vi "Periodic Tasks.vi"(8 "error in":errorcluster) -> ()   [LabVIEW 2013]
doc: "This VI runs in parallel to other tasks. It can contain as many user-defined periodic loops as you need. These can carry out PID or other sorts of timed response."
uses:
  <vilib>/Rock Robotics/SystemInterfaces/Utilities/FPGA_UtilitiesLED Source.ctl
  <vilib>/Rock Robotics/SystemInterfaces/Utilities/FPGA_UtilitiesLED State.ctl
  <vilib>/Rock Robotics/WPI/DriverStation/DriverStationLCD/WPI_DriverStationLCDLCDLine.ctl
  Robot Global Data.vi
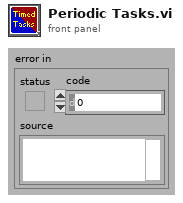
[diagram p1: front panel]
types:
  T1 = typedef "WPI_AnalogChannelDevRef.ctl" = cluster{"DevStatus":errorcluster, "Analog Module":T2, "Analog Channel":T3}
  T2 = typedef "FPGA_TypedefAnalogModule.ctl" = enum16{"Analog Module 1", "Analog Module 2"}
  T3 = typedef "FPGA_AIChannel.ctl" = enum8{"AI 1", "AI 2", "AI 3", "AI 4", "AI 5", "AI 6", "AI 7", "AI 8", "Invalid"}
  T4 = typedef "WPI_DigitalInputDevRef.ctl" = cluster{"DevStatus":errorcluster, "DIO Channel":T5, "Digital Module":T6}
  T5 = typedef "FPGA_DIOChannel.ctl" = enum8{"DIO 1", "DIO 2", "DIO 3", "DIO 4", "DIO 5", "DIO 6", "DIO 7", "DIO 8", "DIO 9", "DIO 10", "DIO 11", "DIO 12", "DIO 13", "DIO 14", "Invalid"}
  T6 = typedef "FPGA_TypedefDigitalModule.ctl" = enum16{"Digital Module 1", "Digital Module 2"}
  T7 = typedef "WPI_EncoderDevRef.ctl" = cluster{"DevStatus":errorcluster, "EncoderIndex":T8, "CounterIndex":T9, "DistancePerCount":dbl, "Decoding Type":T10}
  T8 = typedef "FPGA_EncoderIdx.ctl" = enum8{"Enc 0", "Enc 1", "Enc 2", "Enc 3", "Invalid"}
  T9 = typedef "FPGA_CounterCtrSystemIndex.ctl" = enum8{"Ctr 0", "Ctr 1", "Ctr 2", "Ctr 3", "Ctr 4", "Ctr 5", "Ctr 6", "Ctr 7", "Invalid"}
  T10 = typedef "WPI_EncoderType.ctl" = enum16{"1x", "2x", "4x"}
  T11 = cluster{"Winch Desired Location":dbl, "Winch Desired Location 2":dbl, "Winch Desired Location 3":dbl}
  T12 = typedef "FPGA_UtilitiesLED State.ctl" = enum16{"Off", "On", "Toggle"}
  T13 = typedef "FPGA_UtilitiesLED Source.ctl" = enum16{"User LED", "FPGA LED"}
  T14 = typedef "WPI_DriverStationLCDLCDLine.ctl" = enum16{"Main - Line 1", "User - Line 2", "User - Line 3", "User - Line 4", "User - Line 5", "User - Line 6"}
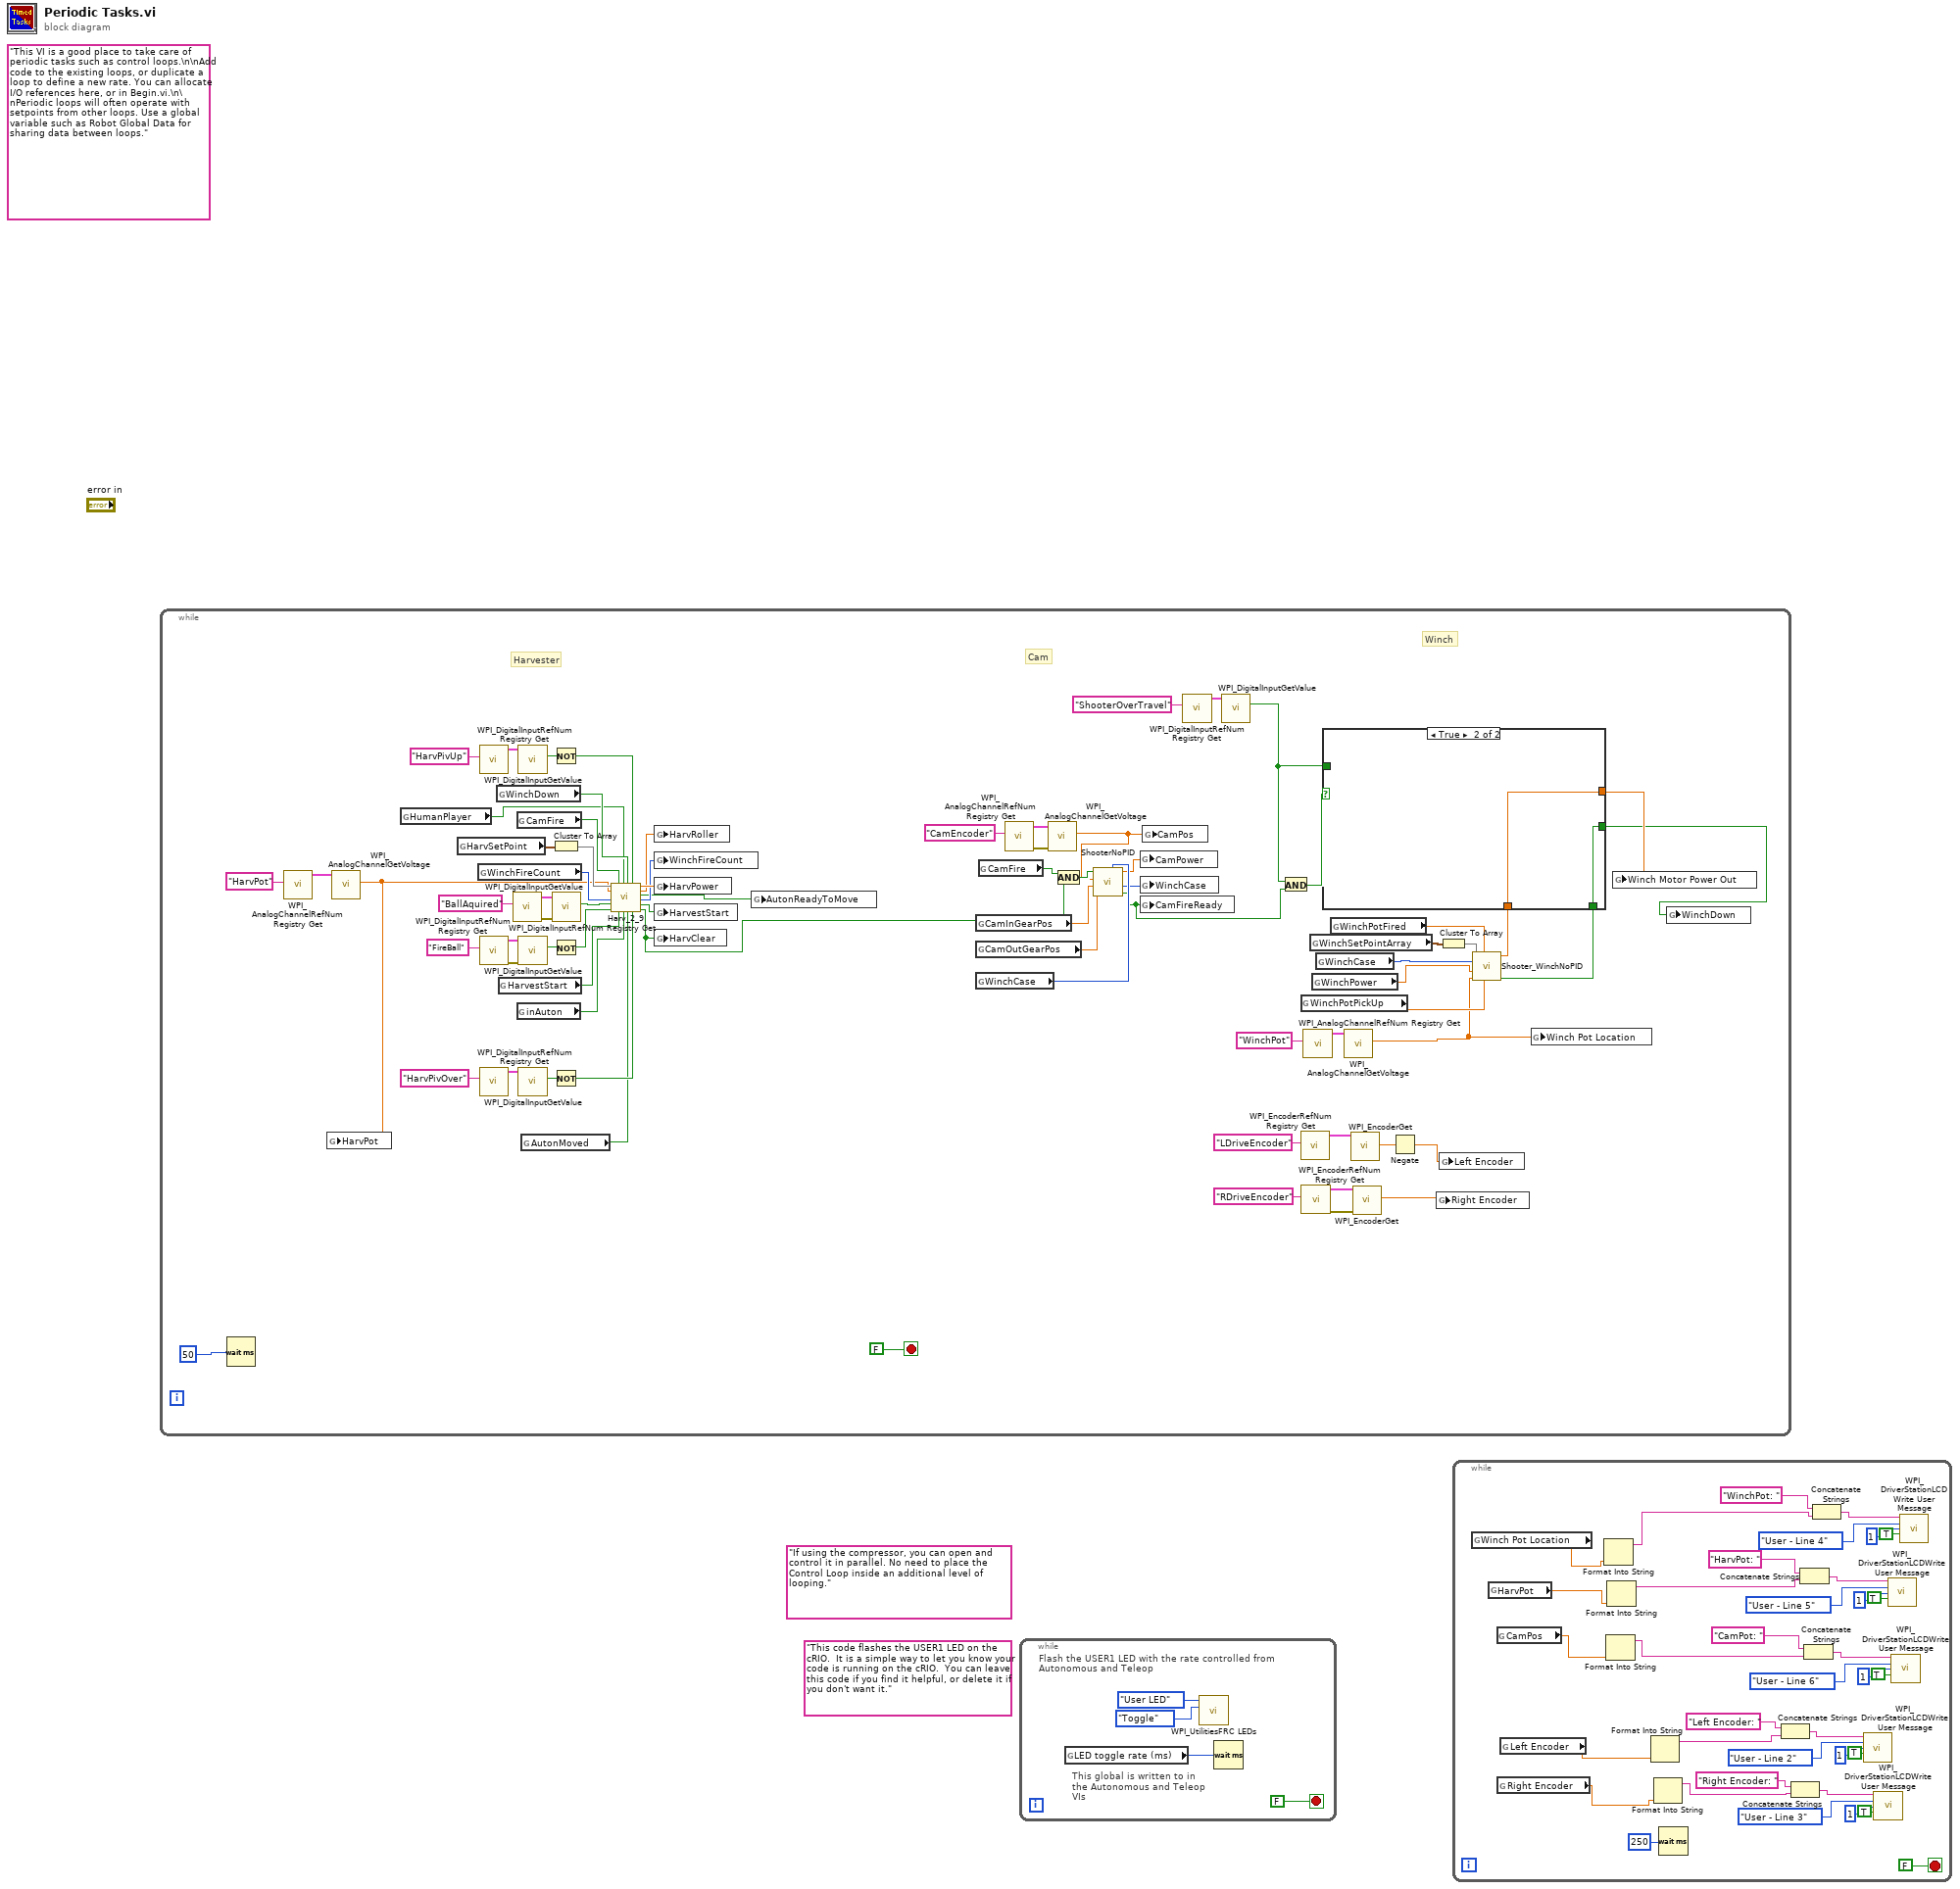
[diagram p0: block diagram]
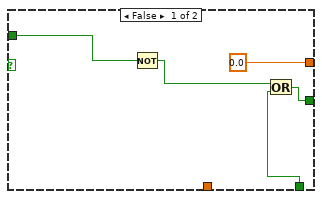
[diagram p2: hidden frame]
diagram:
  (unwired) "If using the compressor, you can open and control it in parallel. No need to place the Control Loop inside an additional level of looping."
  (unwired) "This code flashes the USER1 LED on the cRIO.  It is a simple way to let you know your code is running on the cRIO.  You can leave this code if you find it helpful, or delete it if you don't want it."
  (unwired) "This VI is a good place to take care of periodic tasks such as control loops.\n\nAdd code to the existing loops, or duplicate a loop to define a new rate. You can allocate I/O references here, or in Begin.vi.\n\nPeriodic loops will often operate with setpoints from other loops. Use a global variable such as Robot Global Data for sharing data between loops."
  n1 = while {
    stop <- FALSE stop-if-true
    # "Winch"
    # "Cam"
    # "Harvester"
    n2 = Wait (ms)(milliseconds to wait=u32 50) -> ()  [unwired: 1 out]
    n3 = call <vilib>:"WPI_AnalogChannelRefNum Registry Get.vi"("refnum name"="HarvPot") -> ("AIDeviceRef"=w73:T1)  [unwired: 9 in, 1 out]
    n4 = call <vilib>:"WPI_AnalogChannelGetVoltage.vi"("AIDeviceRef"=w73) -> ("Voltage"=w12:dbl)  [unwired: 8 in, 2 out]
    n5 = global write "Robot Global Data.vi" "HarvPot"(w12) -> ()
    n6 = global read "Robot Global Data.vi" "HumanPlayer"() -> (w3:bool)
    n7 = global read "Robot Global Data.vi" "HarvSetPoint"() -> (w40:cluster{"Out":dbl, "In":dbl, "Clear":dbl})
    n8 = global read "Robot Global Data.vi" "WinchFireCount"() -> (w15:i32)
    n9 = call <vilib>:"WPI_DigitalInputRefNum Registry Get.vi"("refnum name"="HarvPivUp") -> ("DigitalInputDevRef"=w57:T4)  [unwired: 9 in, 1 out]
    n10 = call <vilib>:"WPI_DigitalInputRefNum Registry Get.vi"("refnum name"="FireBall") -> ("error out"=w46:errorcluster, "DigitalInputDevRef"=w47:T4)  [unwired: 9 in]
    n11 = call <vilib>:"WPI_DigitalInputRefNum Registry Get.vi"("refnum name"="HarvPivOver") -> ("DigitalInputDevRef"=w65:T4)  [unwired: 9 in, 1 out]
    n12 = global read "Robot Global Data.vi" "WinchDown"() -> (w33:bool)
    n13 = global read "Robot Global Data.vi" "HarvestStart"() -> (w44:bool)
    n14 = call <vilib>:"WPI_DigitalInputRefNum Registry Get.vi"("refnum name"="BallAquired") -> ("error out"=w53:errorcluster, "DigitalInputDevRef"=w52:T4)  [unwired: 9 in]
    n15 = global read "Robot Global Data.vi" "CamFire"() -> (w45:bool)
    n16 = global read "Robot Global Data.vi" "inAuton"() -> (w17:bool)
    n17 = call <vilib>:"WPI_DigitalInputGetValue.vi"("DigitalInputDevRef"=w57) -> ("Value"=w36:bool)  [unwired: 8 in, 2 out]
    n18 = call <vilib>:"WPI_DigitalInputGetValue.vi"("error in (no error)"=w46, "DigitalInputDevRef"=w47) -> ("Value"=w43:bool)  [unwired: 7 in, 2 out]
    n19 = call <vilib>:"WPI_DigitalInputGetValue.vi"("DigitalInputDevRef"=w65) -> ("Value"=w38:bool)  [unwired: 8 in, 2 out]
    n20 = global read "Robot Global Data.vi" "AutonMoved"() -> (w2:bool)
    n21 = Not(x=w36) -> (.not. x?=w35:bool)
    n22 = Cluster To Array(cluster=w40) -> (array=w39:dbl[])
    n23 = call <vilib>:"WPI_DigitalInputGetValue.vi"("error in (no error)"=w53, "DigitalInputDevRef"=w52) -> ("Value"=w42:bool)  [unwired: 7 in, 2 out]
    n24 = Not(x=w43) -> (.not. x?=w41:bool)
    n25 = Not(x=w38) -> (.not. x?=w37:bool)
    n26 = call "Harv_2_9.vi"("HarvSetpoints"=w39, "HarvPot"=w12, "Count"=w15, "BallAcquired"=w42, "FireBallSen"=w41, "Fire"=w45, "Harvest"=w44, "HPButton"=w3, "inAuton?"=w17, "WinchDown"=w33, "AutonMoved"=w2, "HarvPivUP"=w35, "HarvPivPickupLim"=w37) -> ("HarvPower"=w50:dbl, "HarvRoller"=w49:dbl, "AutonReadyToMove"=w1:bool, "CountOut"=w14:i32, "HarvStart"=w34:bool, "HarvCleared"=w7:bool)  [unwired: 1 in]
    n27 = global write "Robot Global Data.vi" "HarvRoller"(w49) -> ()
    n28 = global write "Robot Global Data.vi" "WinchFireCount"(w14) -> ()
    n29 = global write "Robot Global Data.vi" "HarvPower"(w50) -> ()
    n30 = global write "Robot Global Data.vi" "HarvestStart"(w34) -> ()
    n31 = global write "Robot Global Data.vi" "HarvClear"(w7) -> ()
    n32 = global write "Robot Global Data.vi" "AutonReadyToMove"(w1) -> ()
    n33 = global read "Robot Global Data.vi" "CamInGearPos"() -> (w22:dbl)
    n34 = global read "Robot Global Data.vi" "CamOutGearPos"() -> (w21:dbl)
    n35 = global read "Robot Global Data.vi" "WinchCase"() -> (w23:i32)
    n36 = global read "Robot Global Data.vi" "CamFire"() -> (w59:bool)
    n37 = call <vilib>:"WPI_AnalogChannelRefNum Registry Get.vi"("refnum name"="CamEncoder") -> ("error out"=w61:errorcluster, "AIDeviceRef"=w60:T1)  [unwired: 9 in]
    n38 = call <vilib>:"WPI_AnalogChannelGetVoltage.vi"("error in (no error)"=w61, "AIDeviceRef"=w60) -> ("Voltage"=w11:dbl)  [unwired: 7 in, 2 out]
    n39 = And(x=w59, y=w7) -> (x .and. y?=w24:bool)
    n40 = call "ShooterNoPID.vi"("WinchCaseIn"=w23, "InGearPosLow"=w21, "InGearPosHigh"=w22, "Pot"=w11, "Fire"=w24) -> ("There?"=w18:bool, "WinchCase"=w19:i32, "Power"=w20:dbl)  [unwired: 4 in]
    n41 = global write "Robot Global Data.vi" "CamPower"(w20) -> ()
    n42 = global write "Robot Global Data.vi" "WinchCase"(w19) -> ()
    n43 = global write "Robot Global Data.vi" "CamFireReady"(w18) -> ()
    n44 = global write "Robot Global Data.vi" "CamPos"(w11) -> ()
    n45 = call <vilib>:"WPI_DigitalInputRefNum Registry Get.vi"("refnum name"="ShooterOverTravel") -> ("DigitalInputDevRef"=w56:T4)  [unwired: 9 in, 1 out]
    n46 = call <vilib>:"WPI_DigitalInputGetValue.vi"("DigitalInputDevRef"=w56) -> ("Value"=w32:bool)  [unwired: 8 in, 2 out]
    n47 = And(x=w32, y=w18) -> (x .and. y?=w54:bool)
    n48 = global read "Robot Global Data.vi" "WinchPotPickUp"() -> (w16:dbl)
    n49 = call <vilib>:"WPI_EncoderRefNum Registry Get.vi"("refnum name"="LDriveEncoder") -> ("EncoderDevRef"=w67:T7)  [unwired: 9 in, 1 out]
    n50 = call <vilib>:"WPI_EncoderRefNum Registry Get.vi"("refnum name"="RDriveEncoder") -> ("error out"=w10:errorcluster, "EncoderDevRef"=w9:T7)  [unwired: 9 in]
    n51 = call <vilib>:"WPI_AnalogChannelRefNum Registry Get.vi"("refnum name"="WinchPot") -> ("AIDeviceRef"=w69:T1)  [unwired: 9 in, 1 out]
    n52 = global read "Robot Global Data.vi" "WinchSetPointArray"() -> (w29:T11)
    n53 = global read "Robot Global Data.vi" "WinchPower"() -> (w31:dbl)
    n54 = global read "Robot Global Data.vi" "WinchCase"() -> (w28:i32)
    n55 = global read "Robot Global Data.vi" "WinchPotFired"() -> (w4:dbl)
    n56 = call <vilib>:"WPI_AnalogChannelGetVoltage.vi"("AIDeviceRef"=w69) -> ("Voltage"=w13:dbl)  [unwired: 8 in, 2 out]
    n57 = call <vilib>:"WPI_EncoderGet.vi"("EncoderDevRef"=w67) -> ("Distance"=w6:dbl)  [unwired: 5 in, 5 out]
    n58 = call <vilib>:"WPI_EncoderGet.vi"("error in (no error)"=w10, "EncoderDevRef"=w9) -> ("Distance"=w8:dbl)  [unwired: 4 in, 5 out]
    n59 = Negate(x=w6) -> (-x=w5:dbl)
    n60 = global write "Robot Global Data.vi" "Right Encoder"(w8) -> ()
    n61 = Cluster To Array(cluster=w29) -> (array=w30:dbl[])
    n62 = global write "Robot Global Data.vi" "Left Encoder"(w5) -> ()
    n63 = call "Shooter_WinchNoPID.vi"("PickStartPos"=w16, "WinchFiredPos"=w4, "Winch Pot Location"=w13, "WinchPower"=w31, "selectedCase"=w28, "SetPointArray"=w30) -> ("isThere?"=w26:bool, "Winch Motor Power Out"=w25:dbl)  [unwired: 4 in]
    n64 = case shown="True" w54 {
      tunnel: [0.0 ("Winch Motor Power Out") w80] -> w63
      tunnel: [w78 w81] -> w27
      tunnel: w32 -> [w77 _]
      tunnel: w26 -> [w75 w81]
      tunnel: w25 -> [_ w80]
      frame False {
        n65 = Not(x=w77) -> (.not. x?=w76:bool)
        n66 = Or(x=w76, y=w75) -> (x .or. y?=w78:bool)
      }
      frame True {
      }
    }
    n67 = global write "Robot Global Data.vi" "Winch Pot Location"(w13) -> ()
    n68 = global write "Robot Global Data.vi" "Winch Motor Power Out"(w63) -> ()
    n69 = global write "Robot Global Data.vi" "WinchDown"(w27) -> ()
  }
  n70 = while {
    stop <- FALSE stop-if-true
    # "This global is written to in the Autonomous and Teleop VIs"
    # "Flash the USER1 LED with the rate controlled from Autonomous and Teleop"
    n71 = global read "Robot Global Data.vi" "LED toggle rate (ms)"() -> (w82:u32)
    n72 = call <vilib>:"WPI_UtilitiesFRC LEDs.vi"("State"=FPGA_UtilitiesLED_State."Toggle", "LED Type"=FPGA_UtilitiesLED_Source."User LED") -> ()  [unwired: 1 in, 9 out]
    n73 = Wait (ms)(milliseconds to wait=w82) -> ()  [unwired: 1 out]
  }
  n74 = while {
    stop <- FALSE stop-if-true
    n75 = global read "Robot Global Data.vi" "Winch Pot Location"() -> (w91:dbl)
    n76 = global read "Robot Global Data.vi" "HarvPot"() -> (w90:dbl)
    n77 = global read "Robot Global Data.vi" "CamPos"() -> (w92:dbl)
    n78 = global read "Robot Global Data.vi" "Right Encoder"() -> (w88:dbl)
    n79 = global read "Robot Global Data.vi" "Left Encoder"() -> (w89:dbl)
    n80 = Format Into String(w91) -> (resulting string=w108:string)  [unwired: 3 in, 1 out]
    n81 = Format Into String(w92) -> (resulting string=w93:string)  [unwired: 3 in, 1 out]
    n82 = Format Into String(w90) -> (resulting string=w102:string)  [unwired: 3 in, 1 out]
    n83 = Format Into String(w89) -> (resulting string=w100:string)  [unwired: 3 in, 1 out]
    n84 = Format Into String(w88) -> (resulting string=w99:string)  [unwired: 3 in, 1 out]
    n85 = Wait (ms)(milliseconds to wait=u32 250) -> ()  [unwired: 1 out]
    n86 = Concatenate Strings("Left Encoder: ", w100) -> (w118:string)
    n87 = Concatenate Strings("Right Encoder: ", w99) -> (w117:string)
    n88 = Concatenate Strings("HarvPot: ", w102) -> (w103:string)
    n89 = Concatenate Strings("CamPot: ", w93) -> (w98:string)
    n90 = Concatenate Strings("WinchPot: ", w108) -> (w113:string)
    n91 = call <vilib>:"WPI_DriverStationLCDWrite User Message.vi"("line text"=w118, "line"=WPI_DriverStationLCDLCDLine."User - Line 2", "starting column"=i8 1, "clear line before write (T)"=TRUE) -> ()  [unwired: 1 in, 11 out]
    n92 = call <vilib>:"WPI_DriverStationLCDWrite User Message.vi"("line text"=w117, "line"=WPI_DriverStationLCDLCDLine."User - Line 3", "starting column"=i8 1, "clear line before write (T)"=TRUE) -> ()  [unwired: 1 in, 11 out]
    n93 = call <vilib>:"WPI_DriverStationLCDWrite User Message.vi"("line text"=w103, "line"=WPI_DriverStationLCDLCDLine."User - Line 5", "starting column"=i8 1, "clear line before write (T)"=TRUE) -> ()  [unwired: 1 in, 11 out]
    n94 = call <vilib>:"WPI_DriverStationLCDWrite User Message.vi"("line text"=w98, "line"=WPI_DriverStationLCDLCDLine."User - Line 6", "starting column"=i8 1, "clear line before write (T)"=TRUE) -> ()  [unwired: 1 in, 11 out]
    n95 = call <vilib>:"WPI_DriverStationLCDWrite User Message.vi"("line text"=w113, "line"=WPI_DriverStationLCDLCDLine."User - Line 4", "starting column"=i8 1, "clear line before write (T)"=TRUE) -> ()  [unwired: 1 in, 11 out]
  }
